vi "Pack.vi"(7 "tcp-message-type":T1=enum."cmd", 11 "String":string) -> (3 "TCP Pack":string)   [LabVIEW 2020, in "CSM-TCP-Router.lvlib"]
uses:
  CSM-TCP-Router.lvlib
  typedef/tcp-msg type.ctl
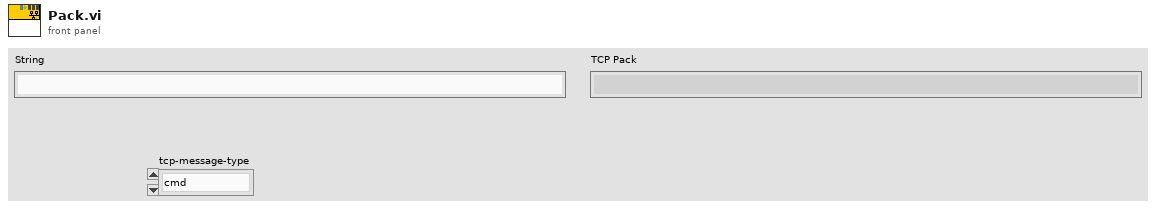
[diagram p1: front panel]
types:
  T1 = typedef "CSM-TCP-Router.lvlib/tcp-msg type.ctl" = enum16{"info", "error", "cmd", "resp", "async-resp", "status", "interrupt"}
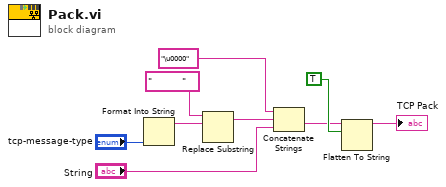
[diagram p0: block diagram]
diagram:
  n1 = Format Into String("tcp-message-type") -> (resulting string=w6:string)  [unwired: 3 in, 1 out]
  n2 = Replace Substring(4:w6, 5:"          ") -> (1:w3:string)  [unwired: 2 in, 1 out]
  n3 = Concatenate Strings("\u0000", w3, "String") -> (w2:string)
  n4 = Flatten To String(anything=w2, prepend array or string size? (T)=TRUE) -> (data string=→"TCP Pack":string)  [unwired: 1 in, 3 out]
